vi "Write8.vi"(8 "error in (no error)":errorcluster, 9 "Data":u8, 10 "Registers":T4, 11 "ColorSensorDevRef":T1={"I2CDevRef"={"DevStatus"={"status"=FALSE, "code"=0, "source"=""}, "Device Address"=0, "Handle"=0, "I2C Bus"=enum."Invalid"}} {"I2CDevRef"."Device Address" format="%.0x"}) -> (0 "error out":errorcluster, 3 "ColorSensorDevRef out":T1={"I2CDevRef"={"DevStatus"={"status"=FALSE, "code"=0, "source"=""}, "Device Address"=0, "Handle"=0, "I2C Bus"=enum."Invalid"}} {"I2CDevRef"."Device Address" format="%.0x"})   [LabVIEW 2018, in "ColorSensor.lvlib"]
uses:
  ColorSensor.lvlib
  ColorSensorDevRef.ctl
  <vilib>/Rock Robotics/WPI/I2C/WPI_I2CDevRef.ctl
  <vilib>/Rock Robotics/SystemInterfaces/i2clib/i2c_bus.ctl
  Registers.ctl
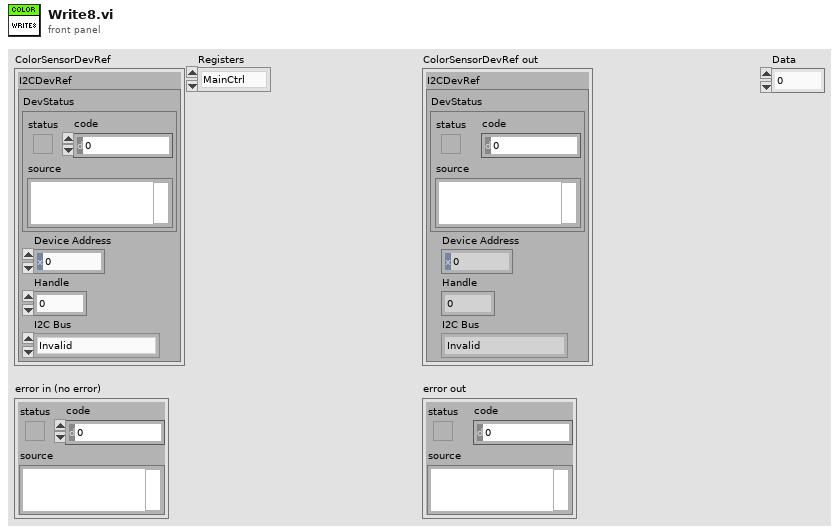
[diagram p1: front panel]
types:
  T1 = typedef "ColorSensor.lvlib/ColorSensorDevRef.ctl" = cluster{"I2CDevRef":T2}
  T2 = typedef "WPI_I2CDevRef.ctl" = cluster{"DevStatus":errorcluster, "Device Address":u8, "Handle":i32, "I2C Bus":T3}
  T3 = typedef "i2c_bus.ctl" = enum16{"I2C On-Board", "I2C MXP", "Invalid"}
  T4 = typedef "ColorSensor.lvlib/Registers.ctl" = enum16{"MainCtrl", "ProximitSensorLED", "ProximitySensorPulse", "ProximitySensorRate", "LightSensorMeasurementRate", "LightSensorGainRegister", "PartIDRegister", "MainStatus", "ProximityData", "ProximityData1", "InfraredData", "InfraredData1", "InfraredData2", "GreenData", "GreenData1", "GreenData2", "BlueData", "BlueData1", "BlueData2", "RedData", "RedData1", "RedData2"}
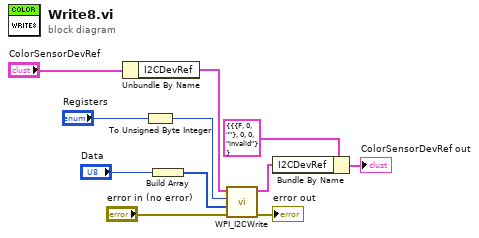
[diagram p0: block diagram]
diagram:
  n1 = Unbundle By Name("ColorSensorDevRef") -> ("I2CDevRef"=w10:T2)
  n2 = To Unsigned Byte Integer(number="Registers") -> (unsigned 8bit integer=w8:u8)
  n3 = Build Array("Data") -> (w1:u8[])
  n4 = call <vilib>:"WPI_I2CWrite.vi"("error in (no error)"="error in (no error)", "I2CDataToSend"=w1, "I2CRegister"=w8, "I2CDevRef"=w10) -> ("error out"=→"error out":errorcluster, "I2CDevRef"=w6:T2)  [unwired: 6 in]
  n5 = Bundle By Name(cluster=T1 {"I2CDevRef"={"DevStatus"={"status"=FALSE, "code"=0, "source"=""}, "Device Address"=0, "Handle"=0, "I2C Bus"=enum."Invalid"}} ("ColorSensorDevRef"), "I2CDevRef"=w6) -> (→"ColorSensorDevRef out":T1)
